vi "advanced 최종.vi"() -> ()   [LabVIEW 2016]
uses:
  <vilib>/DAQmx/write.llb/DAQmx Write (Digital 1D U8 1Chan NSamp).vi
  <vilib>/DAQmx/read.llb/DAQmx Read (Analog 1D Wfm NChan NSamp).vi
  <vilib>/DAQmx/write.llb/DAQmx Write (Analog 1D Wfm NChan NSamp).vi
  <vilib>/DAQmx/create/channels.llb/DAQmx Create Channel (AO-Voltage-Basic).vi
  <vilib>/DAQmx/configure/timing.llb/DAQmx Timing (Sample Clock).vi
  <vilib>/DAQmx/create/channels.llb/DAQmx Create Channel (AI-Voltage-Basic).vi
  <vilib>/DAQmx/create/channels.llb/DAQmx Create Channel (CO-Pulse Generation-Frequency).vi
  <vilib>/DAQmx/configure/timing.llb/DAQmx Timing (Implicit).vi
  <vilib>/DAQmx/configure/trigger.llb/DAQmx Start Trigger (Digital Edge).vi
  <vilib>/DAQmx/create/channels.llb/DAQmx Create Channel (DO-Digital Output).vi
  <vilib>/DAQmx/miscellaneous.llb/DAQmx Fill In Error Info.vi
  <resource>/objmgr/daqmx.rc
  <vilib>/measure/NI_MABase.lvlib
panel:
  in  "data":u8[](array[numeric]) caption="데이터" format="%08b"
  in  "lines":tag="Dev2/port0" caption="라인"
  in  "디지털 클럭 속도":dbl=1000.0 caption="클럭속도" format="%0.2f"
  in  "CO 주파수":dbl=1000.0 format="%0.2f"
  in  "트리거 소스":tag="/Dev2/PFI1"
  in  "counter":tag="Dev2/ctr0" caption="카운터"
  out "동시 AO":waveform(dbl)[](graph)
  in  "signal type 2":T1(ring) caption="신호 타입"
  in  "amplitude 2":dbl=1.0 caption="진폭" format="%0.2p"
  in  "frequency 2":dbl=10.0 caption="주파수" format="%0.2p"
  out "동시 AI":waveform(dbl)[](graph)
  in  "정지":bool
  in  "I/O 크기":dbl=1000.0 caption="크기" format="%0.2f"
  in  "signal type":T1(ring) caption="신호 타입"
  in  "amplitude":dbl=1.0 caption="진폭" format="%0.2p"
  in  "frequency":dbl=10.0 caption="주파수" format="%0.2p"
  in  "샘플 갯수":i32=1000 caption="채널당 샘플"
  in  "Output 속도":dbl=1000.0 format="%0.2f"
  # "카운터 설정 값"
  # "디지털"
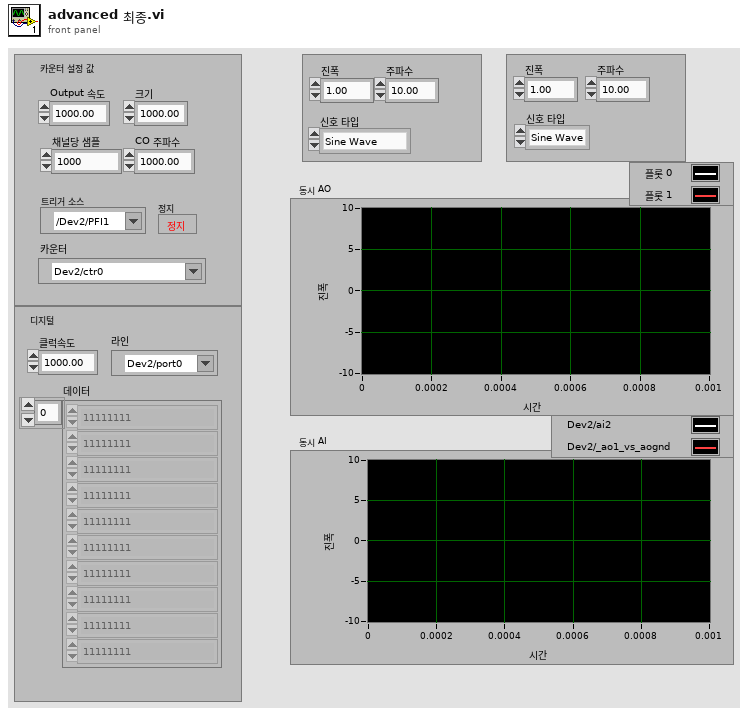
[diagram p1: front panel]
types:
  T1 = enum16{"Sine Wave", "Triangle Wave", "Square Wave", "Sawtooth Wave"}
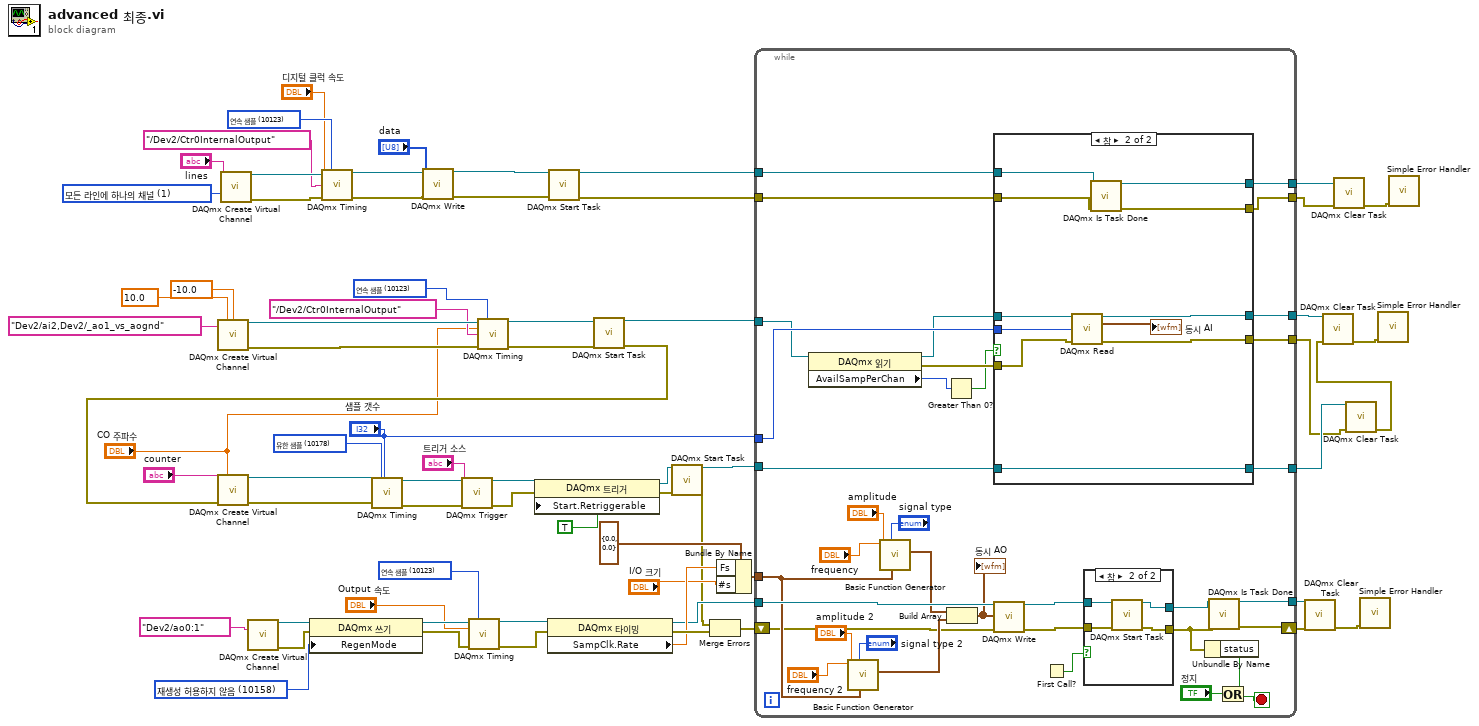
[diagram p0: block diagram]
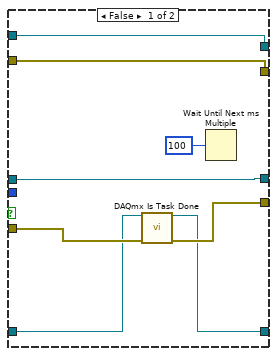
[diagram p2: hidden frame]
diagram:
  w7 = 10123 items=["유한 샘플"=10178, "연속 샘플"=10123, "하드웨어 타이밍에 의한 단일 포인트"=12522] ("sample mode")
  w20 = 1 items=["각 라인에 하나의 채널", "모든 라인에 하나의 채널"] ("line grouping")
  w35 = 10178 items=["유한 샘플"=10178, "연속 샘플"=10123, "하드웨어 타이밍에 의한 단일 포인트"=12522] ("sample mode")
  w40 = 10123 items=["유한 샘플"=10178, "연속 샘플"=10123, "하드웨어 타이밍에 의한 단일 포인트"=12522] ("sample mode")
  w56 = 10123 items=["유한 샘플"=10178, "연속 샘플"=10123, "하드웨어 타이밍에 의한 단일 포인트"=12522] ("sample mode")
  w57 = 10158 items=["재생성 허용"=10097, "재생성 허용하지 않음"=10158] ("재생성 모드")
  n1 = call-poly <vilib>:"DAQmx Create Virtual Channel.vi"("maximum value"=10.0, "minimum value"=-10.0, "physical channels"=tag "Dev2/ai2,Dev2/_ao1_vs_aognd") -> ("task out"=w61:refnum<k21>, "error out"=w69:errorcluster)  [unwired: 11 in]
  n2 = call-poly <vilib>:"DAQmx Create Virtual Channel.vi"("lines"="lines", "line grouping"=w20) -> ("task out"=w18:refnum<k21>, "error out"=w19:errorcluster)  [unwired: 12 in]
  n3 = call-poly <vilib>:"DAQmx Create Virtual Channel.vi"("physical channels"=tag "Dev2/ao0:1") -> ("task out"=w67:refnum<k21>, "error out"=w64:errorcluster)  [unwired: 13 in]
  n4 = property class="DAQmx 쓰기"(reference=w67, error in=w64, "RegenMode"=w57) -> (reference out=w66:refnum<k21>, error out=w63:errorcluster)
  n5 = call-poly <vilib>:"DAQmx Timing.vi"("task/channels in"=w18, "sample mode"=w7, "rate"="디지털 클럭 속도", "source"=tag "/Dev2/Ctr0InternalOutput", "error in"=w19) -> ("task out"=w17:refnum<k21>, "error out"=w16:errorcluster)  [unwired: 9 in]
  n6 = call-poly <vilib>:"DAQmx Write.vi"("task/channels in"=w17, "data"="data", "error in"=w16) -> ("task out"=w15:refnum<k21>, "error out"=w14:errorcluster)  [unwired: 10 in, 1 out]
  n7 = call-poly <vilib>:"DAQmx Timing.vi"("task/channels in"=w66, "sample mode"=w56, "rate"="Output 속도", "error in"=w63) -> ("task out"=w65:refnum<k21>, "error out"=w62:errorcluster)  [unwired: 10 in]
  n8 = call-poly <vilib>:"DAQmx Timing.vi"("task/channels in"=w61, "sample mode"=w40, "rate"="CO 주파수", "source"=tag "/Dev2/Ctr0InternalOutput", "error in"=w69) -> ("task out"=w60:refnum<k21>, "error out"=w68:errorcluster)  [unwired: 9 in]
  n9 = property class="DAQmx 타이밍"(reference=w65, error in=w62) -> (reference out=w49:refnum<k21>, error out=w55:errorcluster, "SampClk.Rate"=w52:dbl)
  n10 = call <vilib>:"DAQmx Start Task.vi"("task/channels in"=w15, "error in"=w14) -> ("task out"=w12:refnum<k21>, "error out"=w13:errorcluster)  [unwired: 12 in]
  n11 = call <vilib>:"DAQmx Start Task.vi"("task/channels in"=w60, "error in"=w68) -> ("task out"=w48:refnum<k21>, "error out"=w33:errorcluster)  [unwired: 12 in]
  n12 = call-poly <vilib>:"DAQmx Create Virtual Channel.vi"("frequency"="CO 주파수", "counter"="counter", "error in"=w33) -> ("task out"=w38:refnum<k21>, "error out"=w37:errorcluster)  [unwired: 11 in]
  n13 = call-poly <vilib>:"DAQmx Timing.vi"("task/channels in"=w38, "sample mode"=w35, "samples per channel"="샘플 갯수", "error in"=w37) -> ("task out"=w32:refnum<k21>, "error out"=w31:errorcluster)  [unwired: 10 in]
  n14 = call-poly <vilib>:"DAQmx Trigger.vi"("task/channels in"=w32, "source"="트리거 소스", "error in"=w31) -> ("task out"=w24:refnum<k21>, "error out"=w29:errorcluster)  [unwired: 11 in]
  n15 = property class="DAQmx 트리거"(reference=w24, error in=w29, "Start.Retriggerable"=TRUE ("시작:추가 옵션:재트리거 가능")) -> (reference out=w26:refnum<k21>, error out=w28:errorcluster)
  n16 = call <vilib>:"DAQmx Start Task.vi"("task/channels in"=w26, "error in"=w28) -> ("task out"=w25:refnum<k21>, "error out"=w27:errorcluster)  [unwired: 12 in]
  n17 = Merge Errors(w27, w55) -> (w54:errorcluster)
  n18 = Bundle By Name(cluster=cluster{"Fs":dbl, "#s":dbl} {"Fs"=0.0, "#s"=0.0} ("sampling info"), "Fs"=w52, "#s"="I/O 크기") -> (w50:cluster{"Fs":dbl, "#s":dbl})
  n19 = while {
    shift-right: [w94] -> w46
    shift-left: w54 -> [w70]
    tunnel: w50 -> [w83]
    tunnel: w49 -> [w102]
    tunnel: w48 -> [w81]
    tunnel: [w92] -> w47
    tunnel: [w91] -> w43
    tunnel: [w90] -> w2
    tunnel: w25 -> [w78]
    tunnel: "샘플 갯수" -> [w82]
    tunnel: w12 -> [w75]
    tunnel: [w72] -> w10
    tunnel: w13 -> [w74]
    tunnel: [w73] -> w9
    tunnel: [w71] -> w3
    stop <- w96 stop-if-true
    n20 = property class="DAQmx 읽기"(reference=w81) -> (reference out=w80:refnum<k21>, error out=w79:errorcluster, "AvailSampPerChan"=w77:u32)  [unwired: 1 in]
    n21 = call <vilib>:"Basic Function Generator.vi"("sampling info"=w83, "signal type"="signal type 2", "amplitude"="amplitude 2", "frequency"="frequency 2") -> ("signal out"=w85:waveform(dbl))  [unwired: 5 in, 2 out]
    n22 = call <vilib>:"Basic Function Generator.vi"("sampling info"=w83, "signal type"="signal type", "amplitude"="amplitude", "frequency"="frequency") -> ("signal out"=w86:waveform(dbl))  [unwired: 5 in, 2 out]
    n23 = Greater Than 0?(x=w77) -> (x > 0?=w76:bool)
    n24 = Build Array(w86, w85) -> (w84:waveform(dbl)[])
    "동시 AO" <- w84
    n25 = case shown="참" w76 {
      tunnel: w80 -> [w106 w124]
      tunnel: [w106 w123] -> w91
      tunnel: [w112 w122] -> w90
      tunnel: w82 -> [_ w120]
      tunnel: w79 -> [w111 w119]
      tunnel: w78 -> [w110 w114]
      tunnel: w75 -> [w109 w118]
      tunnel: w74 -> [w108 w116]
      tunnel: [w109 w117] -> w72
      tunnel: [w108 w115] -> w73
      tunnel: [w107 w114] -> w71
      frame False {
        n26 = call <vilib>:"DAQmx Is Task Done.vi"("task/channels in"=w110, "error in"=w111) -> ("task out"=w107:refnum<k21>, "error out"=w112:errorcluster)  [unwired: 11 in, 1 out]
        n27 = Wait Until Next ms Multiple(millisecond multiple=u32 100 ("대기 시간 (ms)")) -> ()  [unwired: 1 out]
      }
      frame True {
        n28 = call-poly <vilib>:"DAQmx Read.vi"("task/channels in"=w124, "number of samples per channel"=w120, "error in"=w119) -> ("task out"=w123:refnum<k21>, "data"=→"동시 AI":waveform(dbl)[], "error out"=w122:errorcluster)  [unwired: 10 in]
        n29 = call <vilib>:"DAQmx Is Task Done.vi"("task/channels in"=w118, "error in"=w116) -> ("task out"=w117:refnum<k21>, "error out"=w115:errorcluster)  [unwired: 11 in, 1 out]
      }
    }
    n30 = call-poly <vilib>:"DAQmx Write.vi"("task/channels in"=w102, "data"=w84, "error in"=w70) -> ("task out"=w100:refnum<k21>, "error out"=w99:errorcluster)  [unwired: 10 in, 1 out]
    n31 = First Call?() -> (First Call?: T/F=w101:bool)
    n32 = case shown="참" w101 {
      tunnel: [w125 w130] -> w95
      tunnel: [w126 w129] -> w93
      tunnel: w100 -> [w126 w128]
      tunnel: w99 -> [w125 w127]
      frame False {
      }
      frame True {
        n33 = call <vilib>:"DAQmx Start Task.vi"("task/channels in"=w128, "error in"=w127) -> ("task out"=w129:refnum<k21>, "error out"=w130:errorcluster)  [unwired: 12 in]
      }
    }
    n34 = Unbundle By Name(w95) -> ("status"=w98:bool)
    n35 = call <vilib>:"DAQmx Is Task Done.vi"("task/channels in"=w93, "error in"=w95) -> ("task out"=w92:refnum<k21>, "error out"=w94:errorcluster)  [unwired: 11 in, 1 out]
    n36 = Or(x=w98, y="정지") -> (x .or. y?=w96:bool)
  }
  n37 = call <vilib>:"DAQmx Clear Task.vi"("task in"=w47, "error in"=w46) -> ("error out"=w45:errorcluster)  [unwired: 13 in]
  n38 = call <vilib>:"DAQmx Clear Task.vi"("task in"=w10, "error in"=w9) -> ("error out"=w11:errorcluster)  [unwired: 13 in]
  n39 = call <vilib>:"DAQmx Clear Task.vi"("task in"=w3, "error in"=w2) -> ("error out"=w1:errorcluster)  [unwired: 13 in]
  n40 = call <vilib>:"DAQmx Clear Task.vi"("task in"=w43, "error in"=w1) -> ("error out"=w44:errorcluster)  [unwired: 13 in]
  n41 = call <vilib>:"Simple Error Handler.vi"("error in (no error)"=w45) -> ()  [unwired: 4 in, 5 out]
  n42 = call <vilib>:"Simple Error Handler.vi"("error in (no error)"=w44) -> ()  [unwired: 4 in, 5 out]
  n43 = call <vilib>:"Simple Error Handler.vi"("error in (no error)"=w11) -> ()  [unwired: 4 in, 5 out]
